vi "adam-5000-set-DO.vi"(6 "send command":bool, 7 "ack in":string, 8 "error in (no error)":errorcluster, 9 "Output State":bool, 10 "DO Number":u8, 11 "VISA Refnum in":refnum<visa-resource-name>) -> (0 "error out":errorcluster, 1 "success?":bool, 2 "read buffer out":string, 3 "VISA Refnum out":refnum<visa-resource-name>, 4 "Command Used":string, 5 "acknowledge char":string)   [LabVIEW 2024]
panel:
  out "read return":u32
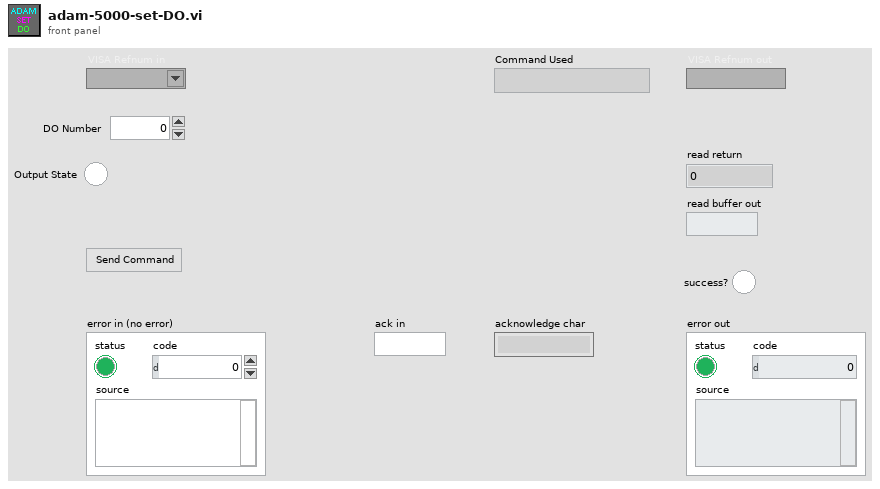
[diagram p1: front panel]
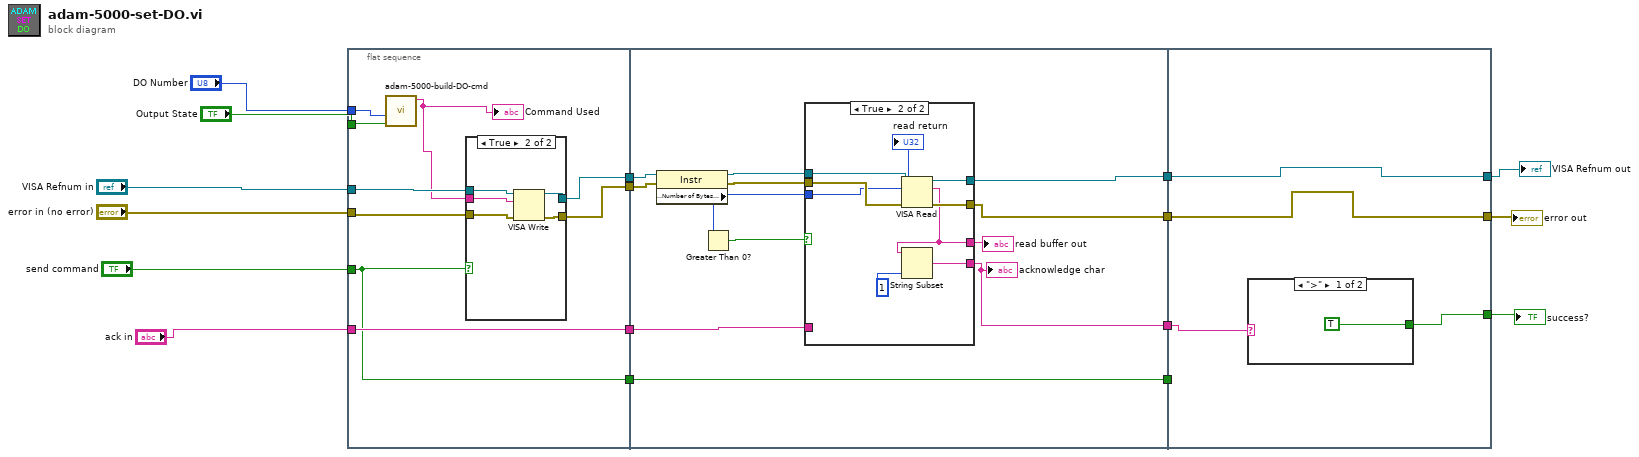
[diagram p0: block diagram]
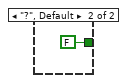
[diagram p4: hidden frame]
diagram:
  n1 = flat-sequence {
    tunnel: "ack in" -> [w26]
    tunnel: "send command" -> [w25]
    tunnel: [w25] -> w12
    tunnel: [w26] -> w11
    tunnel: [w22] -> w10
    tunnel: [w21] -> w9
    tunnel: "VISA Refnum in" -> [w24]
    tunnel: "error in (no error)" -> [w23]
    tunnel: "Output State" -> [w20]
    tunnel: "DO Number" -> [w19]
    tunnel: [w36] -> w15
    tunnel: [w45] -> w14
    tunnel: w12 -> [w45]
    tunnel: w11 -> [w39]
    tunnel: w10 -> [w38]
    tunnel: w9 -> [w37]
    tunnel: [w35] -> w4
    tunnel: [w34] -> w2
    tunnel: [w60] -> w16
    tunnel: w15 -> [w61]
    tunnel: w14 -> [_]
    tunnel: [w59] -> w3
    tunnel: w4 -> [w59]
    tunnel: w2 -> [w58]
    tunnel: [w58] -> w1
    frame #0 {
      n2 = call "adam-5000-build-DO-cmd.vi"("Output State"=w20, "DO Number"=w19) -> ("Command Out"=w18:string)  [unwired: 9 in]
      "Command Used" <- w18
      n3 = case shown="True" w25 {
        tunnel: w24 -> [w28 w33]
        tunnel: w23 -> [w27 w32]
        tunnel: w18 -> [_ w31]
        tunnel: [w28 w30] -> w22
        tunnel: [w27 w29] -> w21
        frame False {
        }
        frame True {
          n4 = VISA Write(VISA resource name=w33, write buffer=w31, error in (no error)=w32) -> (VISA resource name out=w30:refnum<visa-resource-name>, error out=w29:errorcluster)  [unwired: 1 out]
        }
      }
    }
    frame #1 {
      n5 = property class="Instr"(reference=w38, error in=w37) -> (reference out=w42:refnum<visa-resource-name>, error out=w43:errorcluster, "Serial Settings:Number of Bytes at Serial Port"=w41:u32)
      n6 = Greater Than 0?(x=w41) -> (x > 0?=w40:bool)
      n7 = case shown="True" w40 {
        tunnel: w43 -> [w48 w57]
        tunnel: w42 -> [w47 w56]
        tunnel: [w46 w54] -> w36
        tunnel: [w48 w53] -> w34
        tunnel: [w47 w51] -> w35
        tunnel: w41 -> [_ w50]
        tunnel: w39 -> [w46 _]
        tunnel: [w46 w49] -> w44
        frame False {
        }
        frame True {
          n8 = VISA Read(VISA resource name=w56, byte count=w50, error in (no error)=w57) -> (VISA resource name out=w51:refnum<visa-resource-name>, read buffer=w49:string, return count=→"read return":u32, error out=w53:errorcluster)
          n9 = String Subset(string=w49, length (rest)=1 ("length (rest)")) -> (substring=w54:string)  [unwired: 1 in]
        }
      }
      "acknowledge char" <- w36
      "read buffer out" <- w44
    }
    frame #2 {
      n10 = case shown="\">\"" w61 {
        tunnel: [TRUE ("success?") FALSE ("success?")] -> w60
        frame ">" {
        }
        frame "?", Default {
        }
      }
    }
  }
  "success?" <- w16
  "VISA Refnum out" <- w3
  "error out" <- w1
